vi "test_z85.vi"() -> ()   [LabVIEW 2019]
uses:
  zeromq.lvlib
panel:
  out "decode?":bool
  out "encode?":bool
  out "string":string
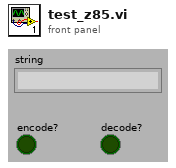
[diagram p1: front panel]
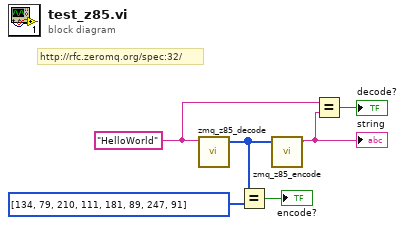
[diagram p0: block diagram]
diagram:
  w3 = "HelloWorld" ("string")
  # "http://rfc.zeromq.org/spec:32/"
  n1 = call "zmq_z85_decode.vi"("encoded string"=w3) -> ("data out"=w5:u8[])  [unwired: 3 in, 1 out]
  n2 = Equal?(x=w5, y=u8[] [134, 79, 210, 111, 181, 89, 247, 91]) -> (x = y?=→"encode?":bool)
  n3 = call "zmq_z85_encode.vi"("data in"=w5) -> ("encoded string"=w2:string)  [unwired: 3 in, 1 out]
  "string" <- w2
  n4 = Equal?(x=w3, y=w2) -> (x = y?=→"decode?":bool)
